vi "Open and Disable Source Separation (Library).vi"(8 "Error In":errorcluster, 11 "Library Path":path) -> (0 "Error Out":errorcluster)   [LabVIEW 2014]
doc: "Copyright (c) 2018 Sze Howe Koh\n\nThis Source Code Form is subject to the terms of the Mozilla Public License, v. 2.0. If a copy of the MPL was not distributed with this file, You can obtain one at http://mozilla.org/MPL/2.0/."
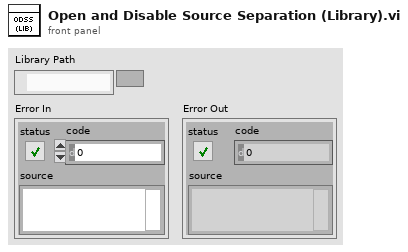
[diagram p1: front panel]
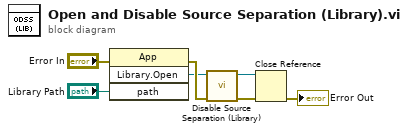
[diagram p0: block diagram]
diagram:
  n1 = invoke class="App" method="Library.Open"(error in="Error In", "path"="Library Path") -> (error out=w7:errorcluster, "Open Library"=w6:refnum<vi>)  [unwired: 2 in, 2 out]
  n2 = call "Disable Source Separation (Library).vi"("Error In"=w7, "Library"=w6) -> ("Error Out"=w1:errorcluster, "Modded Library"=w5:refnum<vi>)  [unwired: 8 in]
  n3 = Close Reference(reference=w5, error in (no error)=w1) -> (error out=→"Error Out":errorcluster)
